vi "SetOutputCurrent.vi"(8 "error in (no error)":errorcluster, 10 "Current":dbl, 11 "RMXPowerSupply in":refnum<class "RMXPowerSupply.lvclass">) -> (0 "error out":errorcluster, 3 "RMXPowerSupply out":refnum<class "RMXPowerSupply.lvclass">)   [LabVIEW 2023, in "RMXPowerSupply.lvclass"]
uses:
  RMXPowerSupply.lvclass
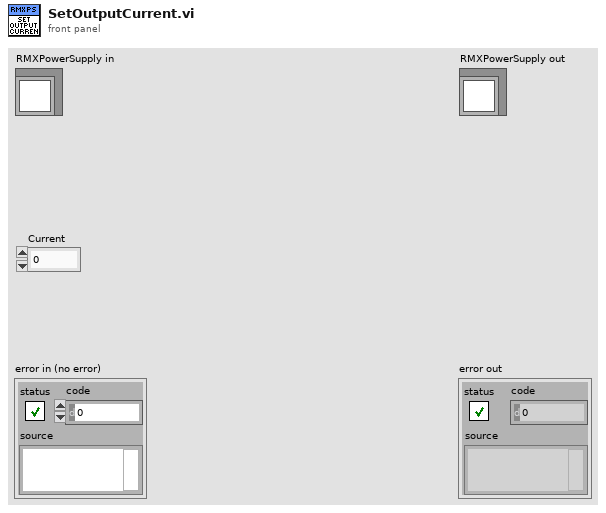
[diagram p1: front panel]
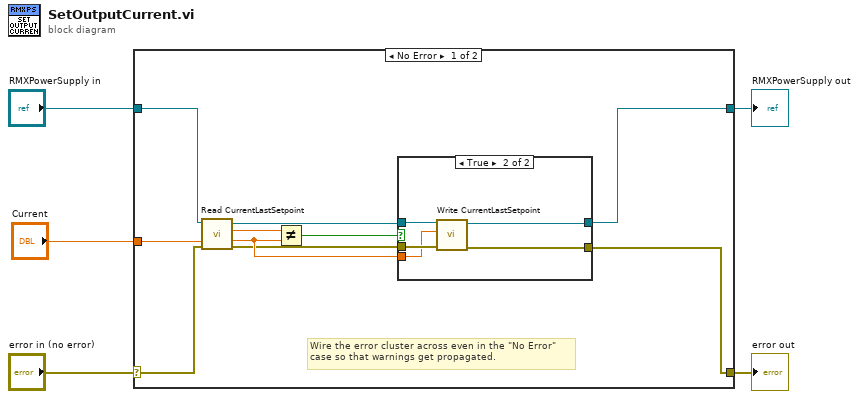
[diagram p0: block diagram]
diagram:
  n1 = case shown="No Error" "error in (no error)" {
    selector: "error in (no error)" -> [w13 w23]
    tunnel: [w6 w23] -> w4
    tunnel: [w7 w22] -> w2
    tunnel: "RMXPowerSupply in" -> [w14 w22]
    tunnel: "Current" -> [w10 _]
    frame No Error {
      # "Wire the error cluster across even in the \"No Error\"\ncase so that warnings get propagated."
      n2 = call-dynamic "Read CurrentLastSetpoint.vi"("error in (no error)"=w13, "RMXPowerSupply in"=w14) -> ("error out"=w9:errorcluster, "CurrentLastSetpoint"=w12:dbl, "RMXPowerSupply out"=w8:refnum<class "RMXPowerSupply.lvclass">)  [unwired: 7 in]
      n3 = Not Equal?(x=w12, y=w10) -> (x != y?=w11:bool)
      n4 = case shown="True" w11 {
        tunnel: w10 -> [_ w17]
        tunnel: w9 -> [w16 w21]
        tunnel: w8 -> [w15 w20]
        tunnel: [w16 w19] -> w6
        tunnel: [w15 w18] -> w7
        frame False {
        }
        frame True {
          n5 = call-dynamic "Write CurrentLastSetpoint.vi"("error in (no error)"=w21, "CurrentLastSetpoint"=w17, "RMXPowerSupply in"=w20) -> ("error out"=w19:errorcluster, "RMXPowerSupply out"=w18:refnum<class "RMXPowerSupply.lvclass">)  [unwired: 7 in]
        }
      }
    }
    frame Error {
    }
  }
  "error out" <- w4
  "RMXPowerSupply out" <- w2
